vi "Put_it.vi"(8 "error in (no error) 2":errorcluster, 10 "Camera Image":T1) -> (0 "error out":errorcluster, 2 "Done":bool)   [LabVIEW 2019]
uses:
  <vilib>/vision/Image Controls.llb/IMAQ Image.ctl
  Mashina_podyehala.vi
  Camera_angle.vi
  Arm_stage_var.vi
  Timer.vi
  <vilib>/vision/NI_Vision_Development_Module.lvlib
  Simulated Robot/Simulation SubVIs/Simulation SubVIs.lvlib
panel:
  out "Stage":i32
  out "New Image":T1
  out "Threshold":T1(plugin-control)
  out "Raw Image":T1(plugin-control)
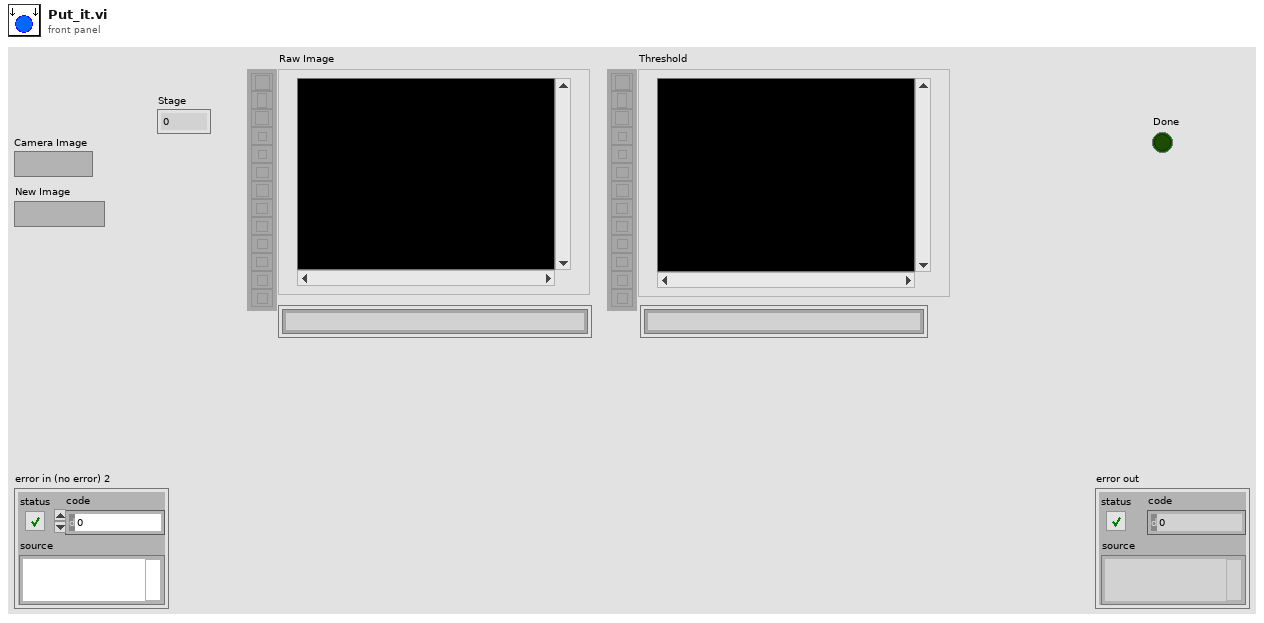
[diagram p1: front panel]
types:
  T1 = typedef "IMAQ Image.ctl" = refnum<image>
  T2 = typedef "Image Type" = u32
  T3 = typedef "Particle Parameters" = i32
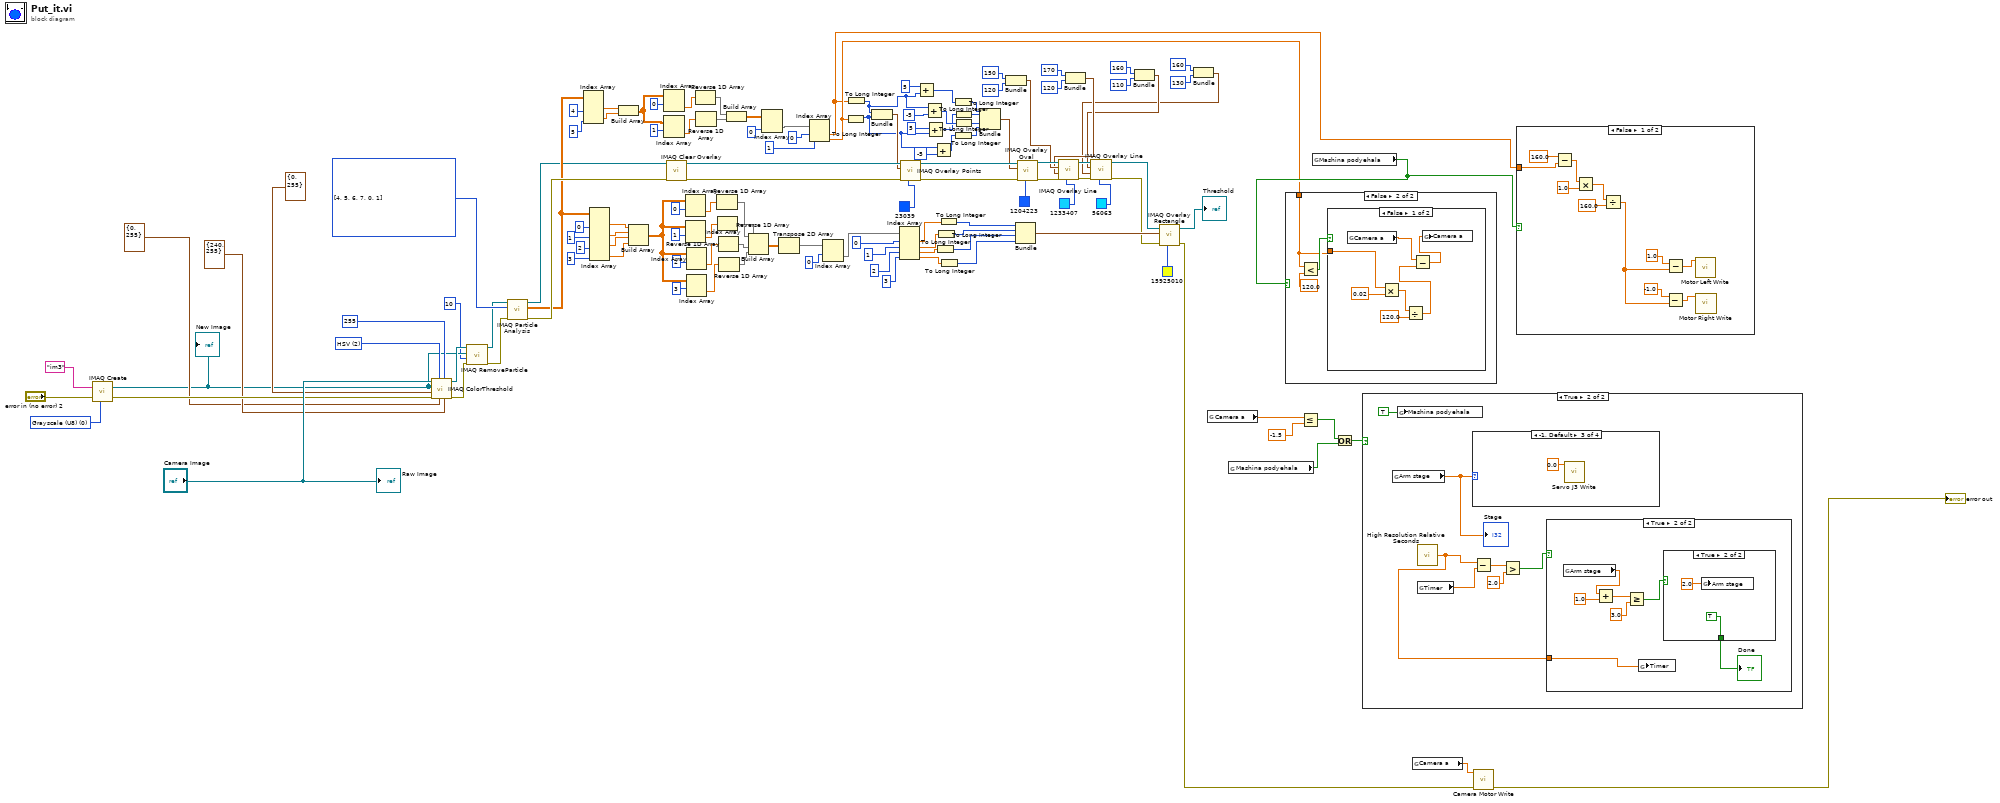
[diagram p0: block diagram]
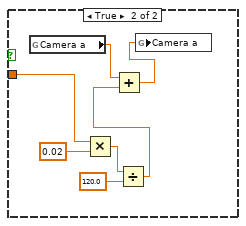
[diagram p3: hidden frame]
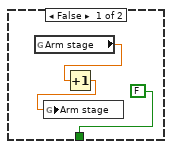
[diagram p6: hidden frame]
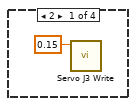
[diagram p7: hidden frame]
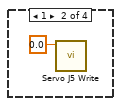
[diagram p8: hidden frame]
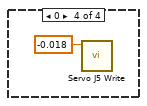
[diagram p9: hidden frame]
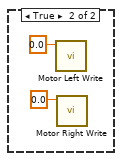
[diagram p10: hidden frame]
diagram:
  w24 = T2 0 items=["Grayscale (U8)", "Grayscale (I16)", "Grayscale (SGL)", "Complex (CSG)", "RGB (U32)", "HSL (U32)", "RGB (U64)", "Grayscale (U16)"] ("Image Type")
  w129 = u16 2 items=["RGB", "HSL", "HSV", "HSI"] ("Color Mode")
  w127 = T3[] [4, 5, 6, 7, 0, 1] items=["Center of Mass X", "Center of Mass Y", "First Pixel X", "First Pixel Y", "Bounding Rect Left", "Bounding Rect Top", "Bounding Rect Right", "Bounding Rect Bottom", "Max Feret Diameter Start X", "Max Feret Diameter Start Y", "Max Feret Diameter End X", "Max Feret Diameter End Y", "Max Horiz. Segment Length Left", "Max Horiz. Segment Length Right", "Max Horiz. Segment Length Row", "-", "Bounding Rect Width", "Bounding Rect Height", "Bounding Rect Diagonal", "Perimeter", "Convex Hull Perimeter", "Holes' Perimeter", "Max Feret Diameter", "Equivalent Ellipse Major Axis", "Equivalent Ellipse Minor Axis", "Equivalent Ellipse Minor Axis (Feret)", "Equivalent Rect Long Side", "Equivalent Rect Short Side", "Equivalent Rect Diagonal", "Equivalent Rect Short Side (Feret)", "Average Horiz. Segment Length", "Average Vert. Segment Length", "Hydraulic Radius", "Waddel Disk Diameter", "-", "Area", "Holes' Area", "Particle & Holes' Area", "Convex Hull Area", "Image Area", "-", "Number of Holes", "Number of Horiz. Segments", "Number of Vert. Segments", "-", "Orientation", "Max Feret Diameter Orientation", "-", "% Area/Image Area", "% Area/(Particle & Holes' Area)", "Ratio of Equivalent Ellipse Axes", "Ratio of Equivalent Rect Sides", "-", "Elongation Factor", "Compactness Factor", "Heywood Circularity Factor", "Type Factor", "-", "Sum X", "Sum Y", "Sum XX", "Sum XY", "Sum YY", "Sum XXX", "Sum XXY", "Sum XYY", "Sum YYY", "-", "Moment of Inertia XX", "Moment of Inertia XY", "Moment of Inertia YY", "Moment of Inertia XXX", "Moment of Inertia XXY", "Moment of Inertia XYY", "Moment of Inertia YYY", "Norm. Moment of Inertia XX", "Norm. Moment of Inertia XY", "Norm. Moment of Inertia YY", "Norm. Moment of Inertia XXX", "Norm. Moment of Inertia XXY", "Norm. Moment of Inertia XYY", "Norm. Moment of Inertia YYY", "Hu Moment 1", "Hu Moment 2", "Hu Moment 3", "Hu Moment 4", "Hu Moment 5", "Hu Moment 6", "Hu Moment 7"] ("Pixel Measurements")
  n1 = call "IMAQ Create"("Image Name"="im3", "Image Type"=w24, "error in (no error)"="error in (no error) 2") -> ("New Image"=w14:T1, "error out"=w22:errorcluster)  [unwired: 2 in]
  "New Image" <- w14
  n2 = call "IMAQ ColorThreshold"("Blue or Luma or Val or Inten Range"=cluster{"Lower value":i32, "Upper value":i32} {"Lower value"=240, "Upper value"=255}, "Replace Value"=255, "Green or Sat Range"=cluster{"Lower value":i32, "Upper value":i32} {"Lower value"=0, "Upper value"=255}, "Color Mode"=w129, "error in (no error)"=w22, "Red or Hue Range"=cluster{"Lower value":i32, "Upper value":i32} {"Lower value"=0, "Upper value"=255}, "Image Dst"=w14, "Image Src"="Camera Image") -> ("error out"=w16:errorcluster, "Image Dst Out"=w17:T1)  [unwired: 2 in]
  n3 = call "IMAQ RemoveParticle"("error in (no error)"=w16, "Number of Erosion"=10, "Image Dst"=w14, "Image Src"=w17) -> ("error out"=w15:errorcluster, "Image Dst Out"=w12:T1)  [unwired: 6 in]
  n4 = call "IMAQ Particle Analysis"("error in (no error)"=w15, "Pixel Measurements"=w127, "Image"=w12) -> ("error out"=w28:errorcluster, "Particle Measurements (Pixels)"=w27:dbl[][], "Image Out (duplicate)"=w21:T1)  [unwired: 3 in, 3 out]
  n5 = Index Array(array=w27, index (col) #1=4 ("disabled index (col)"), index (col) #2=5 ("index (col)")) -> (element #1=w77:dbl[], element #2=w76:dbl[])  [unwired: 2 in]
  n6 = Index Array(array=w27, index (col) #1=0 ("disabled index (col)"), index (col) #2=1 ("index (col)"), index (col) #3=2 ("index (col)"), index (col) #4=3 ("index (col)")) -> (element #1=w122:dbl[], element #2=w121:dbl[], element #3=w120:dbl[], element #4=w119:dbl[])  [unwired: 4 in]
  n7 = Build Array(w77, w76) -> (w73:dbl[][])
  n8 = Build Array(w122, w121, w120, w119) -> (w110:dbl[][])
  n9 = Index Array(array=w73, index (row)=0) -> (element=w72:dbl[])  [unwired: 1 in]
  n10 = Index Array(array=w73, index (row)=1) -> (element=w71:dbl[])  [unwired: 1 in]
  n11 = call "IMAQ Clear Overlay"("error in (no error)"=w28, "Image"=w21) -> ("error out"=w66:errorcluster, "Image Out"=w83:T1)  [unwired: 8 in]
  n12 = Index Array(array=w110, index (row)=0) -> (element=w118:dbl[])  [unwired: 1 in]
  n13 = Index Array(array=w110, index (row)=1) -> (element=w117:dbl[])  [unwired: 1 in]
  n14 = Index Array(array=w110, index (row)=2) -> (element=w116:dbl[])  [unwired: 1 in]
  n15 = Index Array(array=w110, index (row)=3) -> (element=w111:dbl[])  [unwired: 1 in]
  n16 = Reverse 1D Array(array=w72) -> (reversed array=w70:dbl[])
  n17 = Reverse 1D Array(array=w71) -> (reversed array=w69:dbl[])
  n18 = Reverse 1D Array(array=w118) -> (reversed array=w114:dbl[])
  n19 = Reverse 1D Array(array=w117) -> (reversed array=w115:dbl[])
  n20 = Reverse 1D Array(array=w116) -> (reversed array=w113:dbl[])
  n21 = Reverse 1D Array(array=w111) -> (reversed array=w112:dbl[])
  n22 = Build Array(w70, w69) -> (w68:dbl[][])
  n23 = Build Array(w114, w115, w113, w112) -> (w105:dbl[][])
  n24 = Index Array(array=w68, index (col)=0 ("index (row)")) -> (element=w82:dbl[])  [unwired: 1 in]
  n25 = Transpose 2D Array(2D array=w105) -> (transposed array=w93:dbl[][])
  n26 = Index Array(array=w82, index #1=0 ("index"), index #2=1 ("index")) -> (element #1=w4:dbl, element #2=w5:dbl)
  n27 = Index Array(array=w93, index (row)=0) -> (element=w92:dbl[])  [unwired: 1 in]
  n28 = To Long Integer(number=w5) -> (32bit integer=w52:i32)
  n29 = To Long Integer(number=w4) -> (32bit integer=w55:i32)
  n30 = Bundle(w55, w52) -> (w78:cluster{i32, i32})  [unwired: 1 in]
  n31 = Index Array(array=w92, index #1=0 ("index"), index #2=1 ("index"), index #3=2 ("index"), index #4=3 ("index")) -> (element #1=w91:dbl, element #2=w90:dbl, element #3=w89:dbl, element #4=w88:dbl)
  n32 = call "IMAQ Overlay Points"("Color"=u32 23039, "error in (no error)"=w66, "Point"=w78, "Image"=w83) -> ("error out"=w65:errorcluster, "Image Out"=w67:T1)  [unwired: 6 in]
  n33 = Add(x=5, y=w55) -> (x+y=w57:i32)
  n34 = Add(x=w55, y=-5) -> (x+y=w56:i32)
  n35 = Add(x=5, y=w52) -> (x+y=w49:i32)
  n36 = Add(x=w52, y=-5) -> (x+y=w50:i32)
  n37 = To Long Integer(number=w89) -> (32bit integer=w96:i32)
  n38 = To Long Integer(number=w90) -> (32bit integer=w97:i32)
  n39 = To Long Integer(number=w91) -> (32bit integer=w98:i32)
  n40 = To Long Integer(number=w88) -> (32bit integer=w95:i32)
  n41 = To Long Integer(number=w57) -> (32bit integer=w59:i32)
  n42 = To Long Integer(number=w50) -> (32bit integer=w60:i32)
  n43 = To Long Integer(number=w49) -> (32bit integer=w62:i32)
  n44 = To Long Integer(number=w56) -> (32bit integer=w61:i32)
  n45 = Bundle(w59, w62, w61, w60) -> (w63:cluster{i32, i32, i32, i32})  [unwired: 1 in]
  n46 = Bundle(150, 120) -> (w38:cluster{i32, i32})  [unwired: 1 in]
  n47 = Bundle(w98, w97, w96, w95) -> (w99:cluster{i32, i32, i32, i32})  [unwired: 1 in]
  n48 = call "IMAQ Overlay Oval"("Color"=u32 1204223, "error in (no error)"=w65, "Bounding Rectangle"=w63, "Image"=w67) -> ("error out"=w47:errorcluster, "Image Out"=w48:T1)  [unwired: 6 in]
  n49 = Bundle(170, 120) -> (w35:cluster{i32, i32})  [unwired: 1 in]
  n50 = call "IMAQ Overlay Line"("Color"=u32 1233407, "error in (no error)"=w47, "End Point"=w35, "Start Point"=w38, "Image"=w48) -> ("error out"=w45:errorcluster, "Image Out"=w46:T1)  [unwired: 5 in]
  n51 = Bundle(160, 110) -> (w30:cluster{i32, i32})  [unwired: 1 in]
  n52 = Bundle(160, 130) -> (w29:cluster{i32, i32})  [unwired: 1 in]
  n53 = call "IMAQ Overlay Line"("Color"=u32 56063, "error in (no error)"=w45, "End Point"=w29, "Start Point"=w30, "Image"=w46) -> ("error out"=w44:errorcluster, "Image Out"=w43:T1)  [unwired: 5 in]
  n54 = call "IMAQ Overlay Rectangle"("Color"=u32 15925010, "error in (no error)"=w44, "Rectangle"=w99, "Image"=w43) -> ("error out"=w6:errorcluster, "Image Out"=→"Threshold":T1)  [unwired: 6 in]
  n55 = global read "Camera_angle.vi" "Camera a"() -> (w9:dbl)
  n56 = global read "Mashina_podyehala.vi" "Mashina podyehala"() -> (w1:bool)
  n57 = Less Or Equal?(x=w9, y=-1.5) -> (x <= y?=w2:bool)
  n58 = global read "Mashina_podyehala.vi" "Mashina podyehala"() -> (w10:bool)
  n59 = case shown="False" w10 {
    tunnel: w5 -> [_ w130]
    frame True {
    }
    frame False {
      n60 = Less?(x=w130, y=120.0) -> (x < y?=w131:bool)
      n61 = case shown="False" w131 {
        tunnel: w130 -> [w138 w142]
        frame False {
          n62 = global read "Camera_angle.vi" "Camera a"() -> (w133:dbl)
          n63 = Multiply(x=w138, y=0.02) -> (x*y=w136:dbl)
          n64 = Divide(x=w136, y=120.0) -> (x/y=w135:dbl)
          n65 = Subtract(x=w133, y=w135) -> (x-y=w134:dbl)
          n66 = global write "Camera_angle.vi" "Camera a"(w134) -> ()
        }
        frame True {
          n67 = global read "Camera_angle.vi" "Camera a"() -> (w140:dbl)
          n68 = Multiply(x=w142, y=0.02) -> (x*y=w144:dbl)
          n69 = Divide(x=w144, y=120.0) -> (x/y=w143:dbl)
          n70 = Add(x=w140, y=w143) -> (x+y=w141:dbl)
          n71 = global write "Camera_angle.vi" "Camera a"(w141) -> ()
        }
      }
    }
  }
  n72 = Or(x=w2, y=w1) -> (x .or. y?=w3:bool)
  n73 = case shown="True" w3 {
    frame False {
    }
    frame True {
      n74 = global read "Arm_stage_var.vi" "Arm stage"() -> (w147:dbl)
      "Stage" <- w147
      n75 = global write "Mashina_podyehala.vi" "Mashina podyehala"(TRUE ("Boolean")) -> ()
      n76 = call <vilib>:"High Resolution Relative Seconds.vi"() -> ("relative seconds"=w150:dbl)
      n77 = global read "Timer.vi" "Timer"() -> (w148:dbl)
      n78 = case shown="-1, Default" w147 {
        frame 2 {
          n79 = call "Servo J3 Write.vi"("J3 Position (m)"=0.15) -> ()  [unwired: 10 in, 1 out]
        }
        frame 1 {
          n80 = call "Servo J5 Write.vi"("J5 Position (m)"=0.0) -> ()  [unwired: 10 in, 1 out]
        }
        frame -1, Default {
          n81 = call "Servo J3 Write.vi"("J3 Position (m)"=0.0) -> ()  [unwired: 10 in, 1 out]
        }
        frame 0 {
          n82 = call "Servo J5 Write.vi"("J5 Position (m)"=-0.018) -> ()  [unwired: 10 in, 1 out]
        }
      }
      n83 = Subtract(x=w150, y=w148) -> (x-y=w153:dbl)
      n84 = Greater?(x=w153, y=2.0) -> (0:w151:bool)
      n85 = case shown="True" w151 {
        tunnel: w150 -> [_ w155]
        frame False {
        }
        frame True {
          n86 = global read "Arm_stage_var.vi" "Arm stage"() -> (w156:dbl)
          n87 = Add(x=w156, y=1.0) -> (x+y=w159:dbl)
          n88 = Greater Or Equal?(x=w159, y=3.0) -> (x >= y?=w158:bool)
          n89 = global write "Timer.vi" "Timer"(w155) -> ()
          n90 = case shown="True" w158 {
            tunnel: [FALSE ("Done") TRUE ("Done")] -> w154
            frame False {
              n91 = global read "Arm_stage_var.vi" "Arm stage"() -> (w163:dbl)
              n92 = Increment(x=w163) -> (x+1=w162:dbl)
              n93 = global write "Arm_stage_var.vi" "Arm stage"(w162) -> ()
            }
            frame True {
              n94 = global write "Arm_stage_var.vi" "Arm stage"(2.0 ("Numeric")) -> ()
            }
          }
          "Done" <- w154
        }
      }
    }
  }
  n95 = global read "Camera_angle.vi" "Camera a"() -> (w8:dbl)
  n96 = call "Camera Motor Write.vi"("error in (no error)"=w6, "Camera Position (rad)"=w8) -> ("error out"=→"error out":errorcluster)  [unwired: 9 in]
  n97 = case shown="False" w10 {
    tunnel: w4 -> [w171 _]
    frame False {
      n98 = Subtract(x=160.0, y=w171) -> (x-y=w170:dbl)
      n99 = Multiply(x=w170, y=1.0) -> (x*y=w179:dbl)
      n100 = Divide(x=w179, y=160.0) -> (x/y=w180:dbl)
      n101 = Subtract(x=-1.0, y=w180) -> (x-y=w178:dbl)
      n102 = Subtract(x=1.0, y=w180) -> (x-y=w177:dbl)
      n103 = call "Motor Left Write.vi"("left motor ccw velocity (rad/s)"=w177) -> ()  [unwired: 10 in, 1 out]
      n104 = call "Motor Right Write.vi"("right motor ccw velocity (rad/s)"=w178) -> ()  [unwired: 10 in, 1 out]
    }
    frame True {
      n105 = call "Motor Left Write.vi"("left motor ccw velocity (rad/s)"=0.0) -> ()  [unwired: 10 in, 1 out]
      n106 = call "Motor Right Write.vi"("right motor ccw velocity (rad/s)"=0.0) -> ()  [unwired: 10 in, 1 out]
    }
  }
  "Raw Image" <- "Camera Image"
